vi "SET_3rdPartyTemplates.vi"(8 "error in (no error)":errorcluster, 10 "3rd party Templates":T1, 11 "Settings.lvclass in":refnum<class "Settings.lvclass">) -> (0 "error out":errorcluster, 3 "Settings.lvclass out":refnum<class "Settings.lvclass">)   [LabVIEW 2020, in "Settings.lvclass"]
uses:
  Settings.lvclass
  Settings.lvclass/Settings.ctl
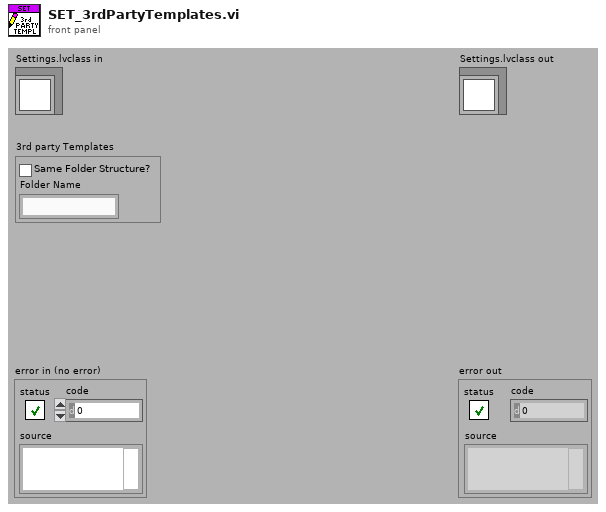
[diagram p1: front panel]
types:
  T1 = cluster{"Same Folder Structure?":bool, "Folder Name":string}
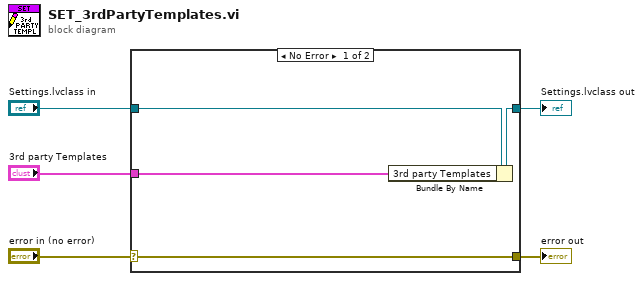
[diagram p0: block diagram]
diagram:
  n1 = case shown="No Error" "error in (no error)" {
    selector: "error in (no error)" -> [w9 w10]
    tunnel: [w9 w10] -> w4
    tunnel: [w7 w11] -> w2
    tunnel: "Settings.lvclass in" -> [w8 w11]
    tunnel: "3rd party Templates" -> [w6 _]
    frame No Error {
      n2 = Bundle By Name(cluster=w8, "3rd party Templates"=w6) -> (w7:refnum<class "Settings.lvclass">)
    }
    frame Error {
    }
  }
  "error out" <- w4
  "Settings.lvclass out" <- w2
